vi "Read Measurement Data (Analog NChan).vi"(0 "VISA resource name":refnum<visa-resource-name>, 5 "Start Channel (1)":string="0001", 7 "End Channel (1)":string="0001", 9 "Data Format (0 : Binary)":i32(ring) items=["Binary", "ASCII"], 11 "error in (no error)":errorcluster) -> (2 "Date Time":timestamp=timestamp(3345116400 s since 1904-01-01) format="%<%H:%M:%S%3u\n%x>T", 4 "VISA resource name out":refnum<visa-resource-name>, 6 "Channel":string[](array[string]), 8 "Data":dbl[](array[numeric]) format="%.4f", 10 "Data Status":i32[](array[ring]) items=["Normal", "Differential Input", "Skip", "Over", "Error", "Burnout", "Power Failure"], 13 "Alarm Status":i32[][](array[ring]) items=["No Alarm", "High Limit Alarm (H)", "Low Limit Alarm (L)", "Difference High Limit Alarm (h)", "Difference Low Limit Alarm (l)", "High Limit on Rate-of-change Alarm (R)", "Low Limit on Rate-of-change Alarm (r)", "Delay High Limit Alarm (T)", "Delay Low Limit Alarm (t)"], 14 "Unit":string[](array[string]), 15 "error out":errorcluster)   [LabVIEW 2020, in "Yokogawa GX Series.lvlib"]
doc: "This VI reads the analog measurement data by ASCII or Binary."
uses:
  <instrlib>/Yokogawa GX Series/Yokogawa GX Series.lvlib
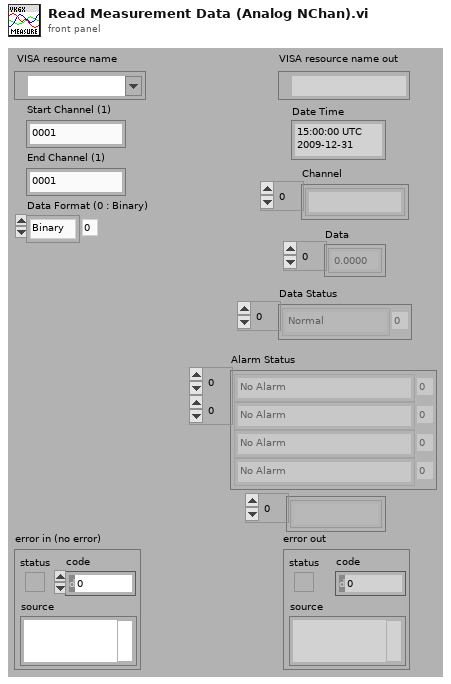
[diagram p1: front panel]
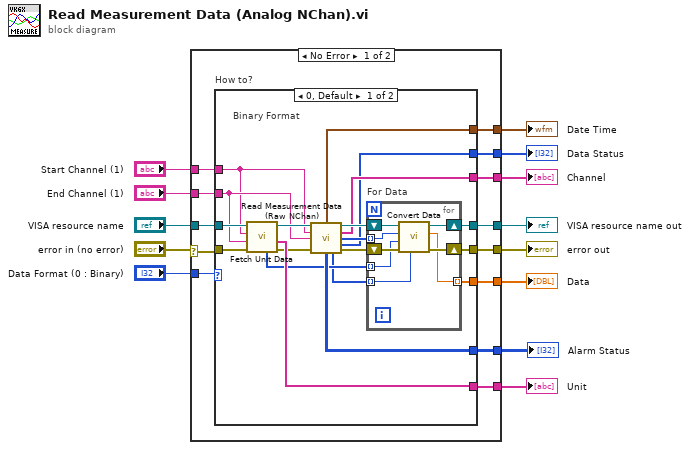
[diagram p0: block diagram]
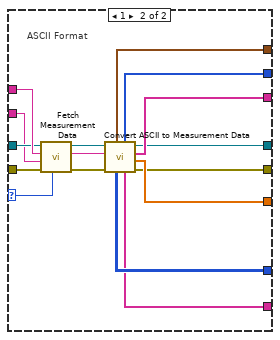
[diagram p2: hidden frame]
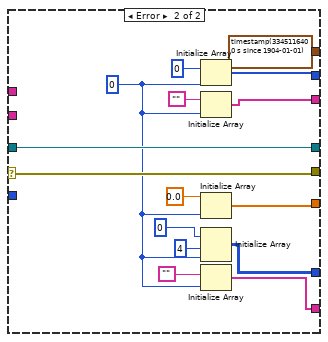
[diagram p3: hidden frame]
diagram:
  n1 = case shown="No Error" "error in (no error)" {
    selector: "error in (no error)" -> [w14 w83]
    tunnel: "VISA resource name" -> [w26 w84]
    tunnel: [w25 w84] -> w12
    tunnel: [w24 w83] -> w11
    tunnel: "Data Format (0 : Binary)" -> [w23 _]
    tunnel: [w22 w74] -> w9
    tunnel: [w21 timestamp(3345116400 s since 1904-01-01)] -> w8
    tunnel: [w20 w78] -> w7
    tunnel: [w19 w77] -> w6
    tunnel: [w18 w70] -> w5
    tunnel: [w17 w81] -> w4
    tunnel: "End Channel (1)" -> [w16 _]
    tunnel: "Start Channel (1)" -> [w15 _]
    frame No Error {
      n2 = case "How to?" shown="0, Default" w23 {
        selector: w23 -> [_ w54]
        tunnel: w26 -> [w34 w68]
        tunnel: w14 -> [w33 w67]
        tunnel: [w45 w57] -> w25
        tunnel: [w44 w60] -> w24
        tunnel: w16 -> [w29 w59]
        tunnel: w15 -> [w28 w69]
        tunnel: [w36 w55] -> w22
        tunnel: [w40 w58] -> w21
        tunnel: [w39 w63] -> w20
        tunnel: [w43 w62] -> w19
        tunnel: [w30 w61] -> w17
        tunnel: [w37 w56] -> w18
        frame 0, Default {
          # "Binary Format"
          n3 = call <instrlib>:"Fetch Unit Data.vi"("error in (no error)"=w33, "End Channel (1)"=w29, "Start Channel (1)"=w28, "VISA resource name"=w34) -> ("error out"=w31:errorcluster, "Unit"=w36:string[], "VISA resource name out"=w32:refnum<visa-resource-name>, "Decimal Position"=w35:i32[])  [unwired: 4 out]
          n4 = call <instrlib>:"Read Measurement Data (Raw NChan).vi"("VISA resource name"=w32, "Start Channel (1)"=w28, "End Channel (1)"=w29, "error in (no error)"=w31) -> ("Date Time"=w40:timestamp, "VISA resource name out"=w42:refnum<visa-resource-name>, "Channel"=w39:string[], "Data"=w38:i32[], "Data Status"=w30:i32[], "Alarm Status"=w37:i32[][], "Data Type"=w27:i32[], "error out"=w41:errorcluster)  [unwired: 4 out]
          n5 = for "For Data" {
            shift-right: [w53] -> w44
            shift-left: w41 -> [w51]
            tunnel: w38 -> [w50] mode=indexing
            tunnel: w35 -> [w47] mode=indexing
            tunnel: [w48] -> w43 mode=indexing
            shift-right: [w52] -> w45
            shift-left: w42 -> [w49]
            tunnel: w27 -> [w46] mode=indexing
            n6 = call <instrlib>:"Convert Data.vi"("Data Type (1 : Int)"=w46, "error in (no error)"=w51, "Decimal Position (0)"=w47, "Integer Data (0)"=w50, "VISA resource name"=w49) -> ("error out"=w53:errorcluster, "Float Data"=w48:dbl, "VISA resource name out"=w52:refnum<visa-resource-name>)  [unwired: 4 out]
          }
        }
        frame 1 {
          # "ASCII Format"
          n7 = call <instrlib>:"Fetch Measurement Data.vi"("Data Format (0 : Binary)"=w54, "error in (no error)"=w67, "End Channel (1)"=w59, "Start Channel (1)"=w69, "VISA resource name"=w68) -> ("error out"=w64:errorcluster, "Measurement Data"=w65:string, "VISA resource name out"=w66:refnum<visa-resource-name>)  [unwired: 4 out]
          n8 = call <instrlib>:"Convert ASCII to Measurement Data.vi"("error in (no error)"=w64, "Measurement ASCII Data (\"\")"=w65, "VISA resource name"=w66) -> ("error out"=w60:errorcluster, "Data"=w62:dbl[], "Channel"=w63:string[], "VISA resource name out"=w57:refnum<visa-resource-name>, "Unit"=w55:string[], "Data Status"=w61:i32[], "Alarm Status"=w56:i32[][], "Date Time"=w58:timestamp)  [unwired: 1 out]
        }
      }
    }
    frame Error {
      w73 = 0
      n9 = Initialize Array(0, w73) -> (w81:i32[])
      n10 = Initialize Array("", w73) -> (w78:string[])
      n11 = Initialize Array(0.0, w73) -> (w77:dbl[])
      n12 = Initialize Array(0, 4, w73) -> (w70:i32[][])
      n13 = Initialize Array("", w73) -> (w74:string[])
    }
  }
  "error out" <- w11
  "VISA resource name out" <- w12
  "Unit" <- w9
  "Channel" <- w7
  "Alarm Status" <- w5
  "Date Time" <- w8
  "Data" <- w6
  "Data Status" <- w4
